vi "ModuloTeste.vi"(0 "IA State Input":T3, 1 "atacando ao contrário?":bool=TRUE, 3 "test module":T1) -> (14 "IA State Output":T3, 15 "ball":dbl(graph), 17 "Robot":dbl(graph))   [LabVIEW 2017]
uses:
  Core/AI Input.ctl
  Core/AI Robot.ctl
  Functions Enum.ctl
  AttackerStates.ctl
  Path Planning/RRT/PathDests.ctl
  Path Planning/RRT/PathDest.ctl
  Core/AI Ball.ctl
  Core/Field Size.ctl
  Core/AI Judge.ctl
  Command Enum.ctl
  Util/Events/Events.ctl
  Test/TestModule.ctl
  Util/Select None or Robot.ctl
  <vilib>/Analysis/_algsub.llb/Real Vector Norm.vi
  <vilib>/Analysis/NI_AALPro.lvlib
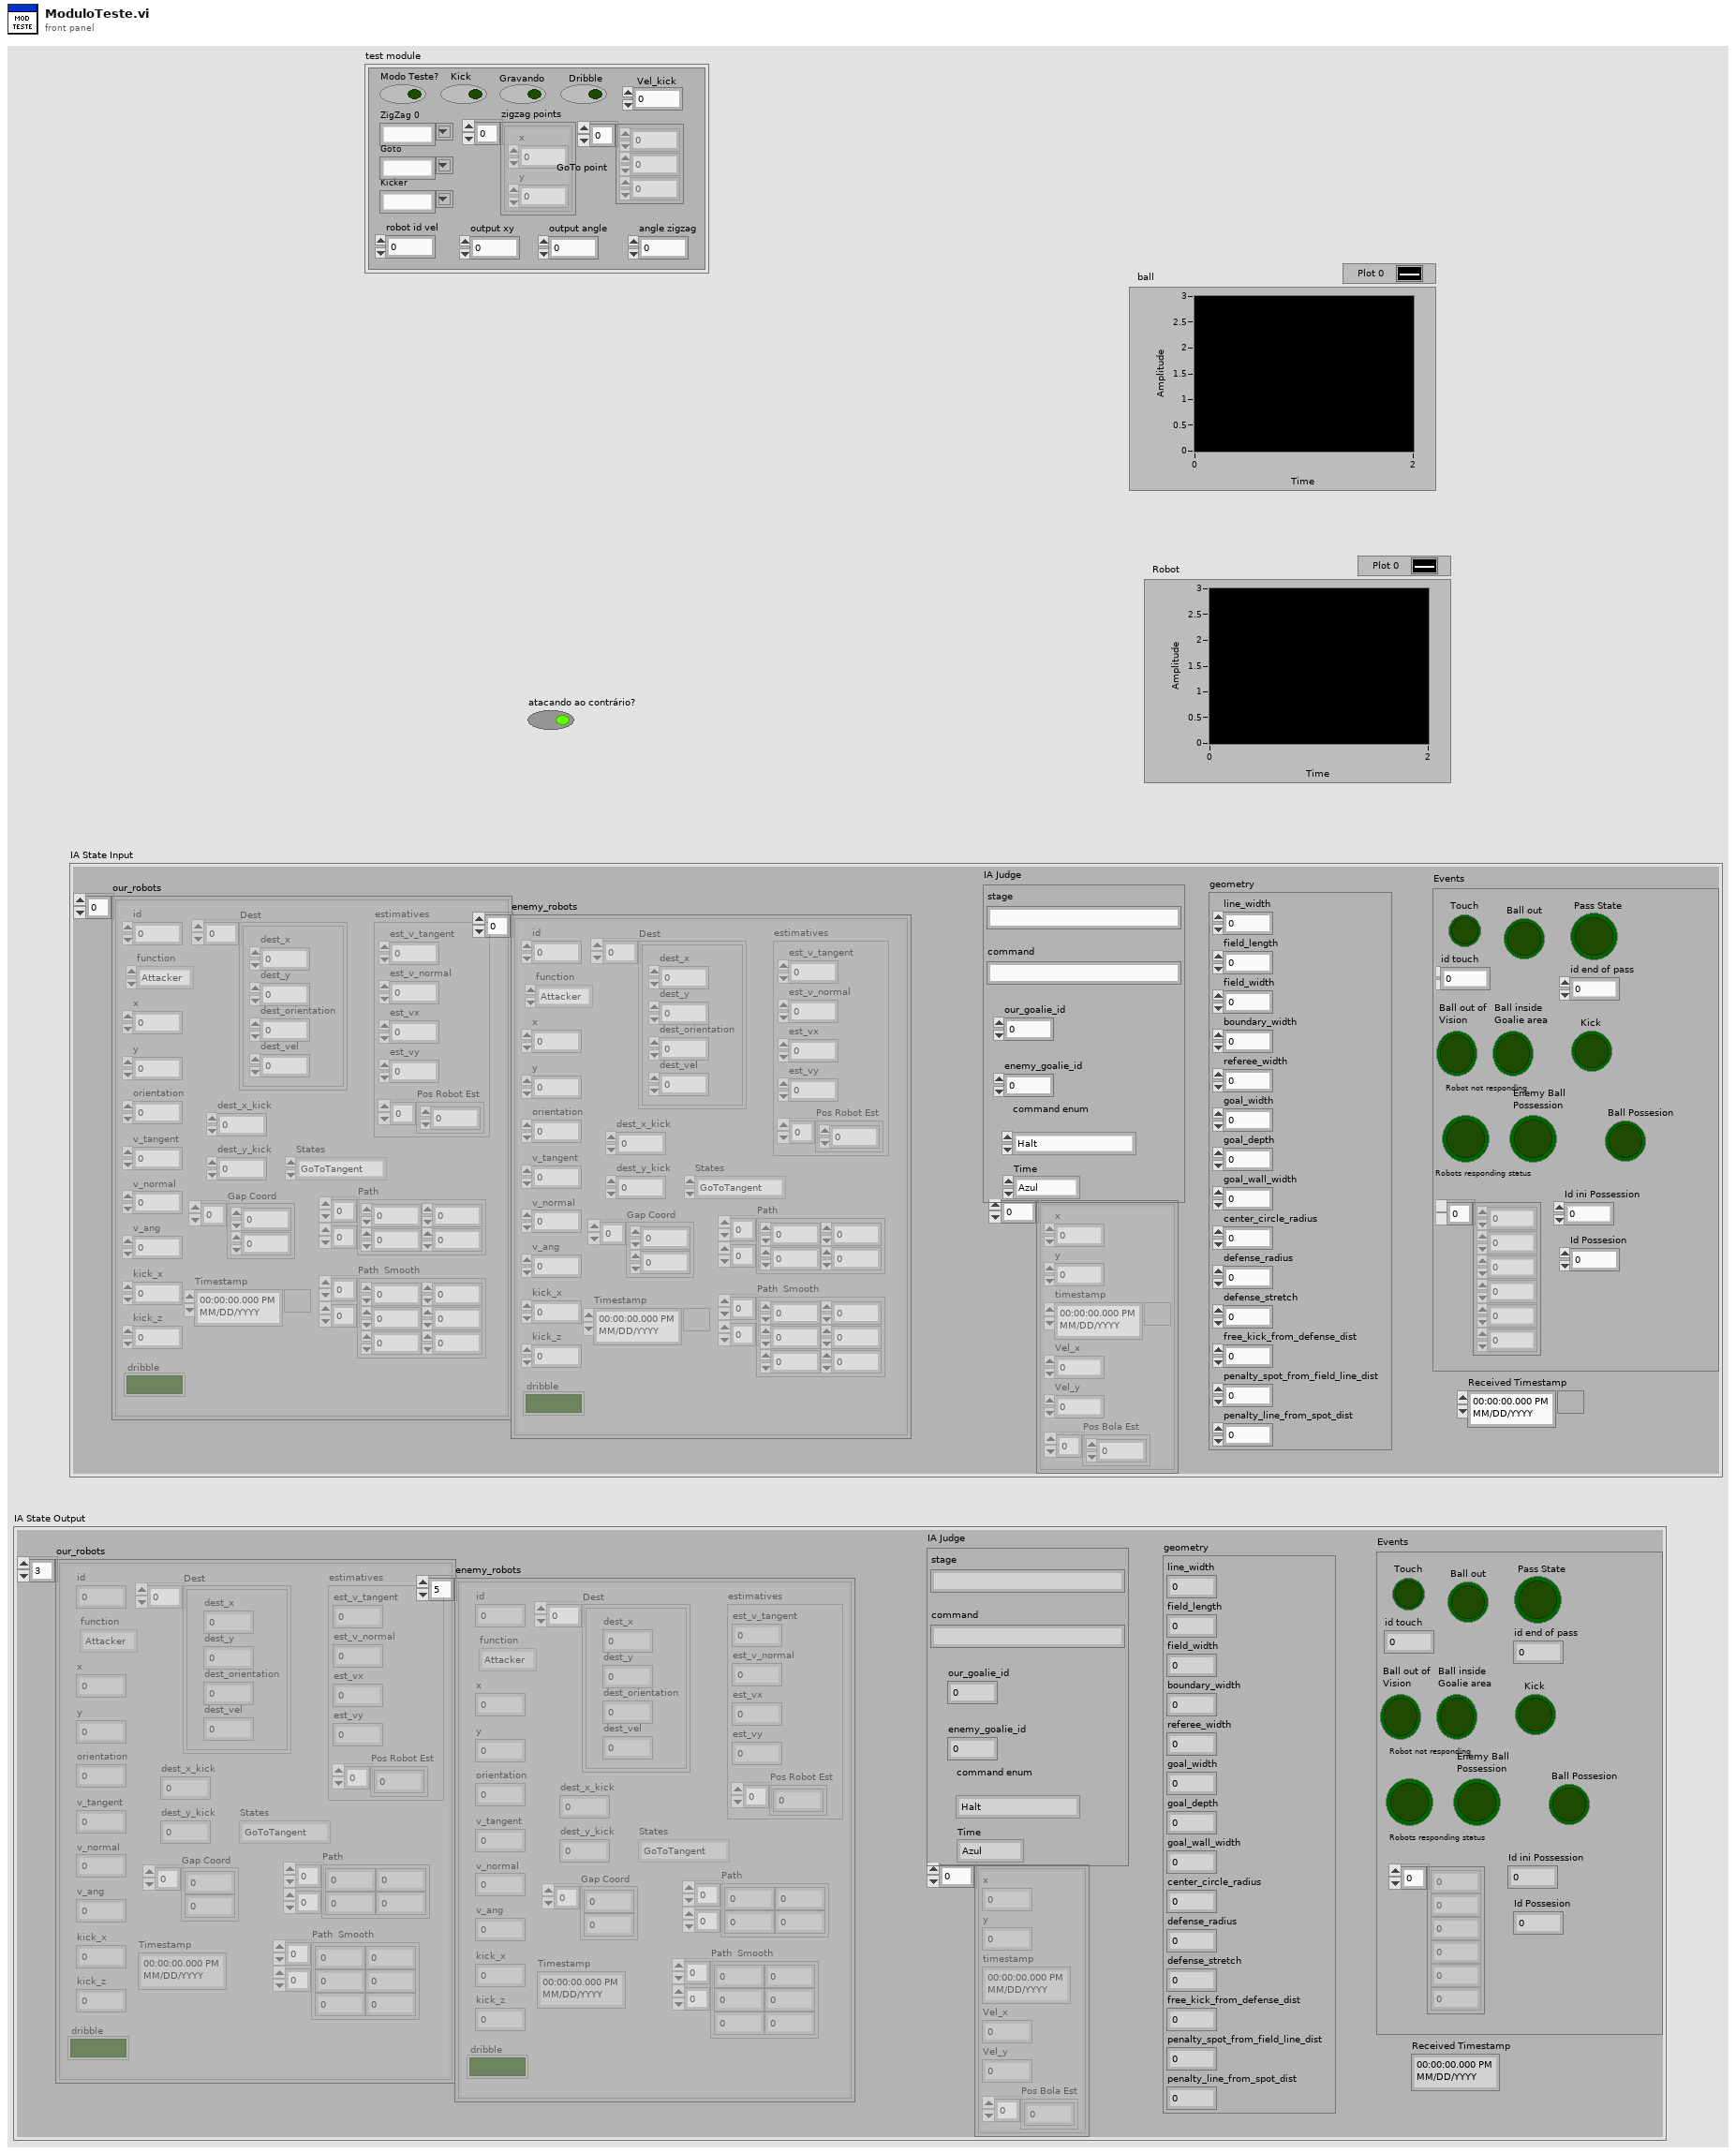
[diagram p1: front panel]
types:
  T1 = typedef "TestModule.ctl" = cluster{"Goto":T2, "ZigZag 0":T2, "Kicker":T2, "Vel_kick":dbl, "Kick":bool, "Modo Teste?":bool, "GoTo point":dbl[], "zigzag points":cluster{"x":dbl, "y":dbl}[], "robot id vel":u32, "Dribble":bool, "Gravando":bool, "output xy":dbl, "output angle":dbl, "angle zigzag":dbl}
  T2 = typedef "Select None or Robot.ctl" = string
  T3 = typedef "AI Input.ctl" = cluster{"our_robots":T4[], "enemy_robots":T4[], "balls":T9[], "geometry":T10, "IA Judge":T11, "Received Timestamp":timestamp, "Events":T13}
  T4 = typedef "AI Robot.ctl" = cluster{"id":u32, "function":T5, "x":dbl, "y":dbl, "orientation":dbl, "v_tangent":dbl, "v_normal":dbl, "v_ang":dbl, "kick_x":dbl, "kick_z":dbl, "dribble":bool, "Timestamp":timestamp, "estimatives":cluster{"est_v_tangent":dbl, "est_v_normal":dbl, "est_vx":dbl, "est_vy":dbl, "Pos Robot Est":dbl[]}, "dest_x_kick":dbl, "dest_y_kick":dbl, "Gap Coord":dbl[], "States":T6, "Path ":dbl[][], "Path  Smooth":dbl[][], "Dest":T7}
  T5 = typedef "Functions Enum.ctl" = enum16{"Attacker", "Goalie", "Defender", "Striker", "Goto 0", "Dummy", "Kicker", "ZigZag"}
  T6 = typedef "AttackerStates.ctl" = enum16{"Pass", "GoToTangent", "BallGetting", "GoToKick", ""}
  T7 = typedef "PathDests.ctl" = T8[]
  T8 = typedef "PathDest.ctl" = cluster{"dest_x":dbl, "dest_y":dbl, "dest_orientation":dbl, "dest_vel":dbl}
  T9 = typedef "AI Ball.ctl" = cluster{"x":dbl, "y":dbl, "timestamp":timestamp, "Vel_x":dbl, "Vel_y":dbl, "Pos Bola Est":dbl[]}
  T10 = typedef "Field Size.ctl" = cluster{"line_width":u32, "field_length":u32, "field_width":u32, "boundary_width":u32, "referee_width":u32, "goal_width":u32, "goal_depth":u32, "goal_wall_width":u32, "center_circle_radius":u32, "defense_radius":u32, "defense_stretch":u32, "free_kick_from_defense_dist":u32, "penalty_spot_from_field_line_dist":u32, "penalty_line_from_spot_dist":u32}
  T11 = typedef "AI Judge.ctl" = cluster{"stage":string, "command":string, "our_goalie_id":dbl, "enemy_goalie_id":dbl, "command enum":T12, "Time":enum16{"Azul", "Amarelo"}}
  T12 = typedef "Command Enum.ctl" = enum16{"Halt", "Stop", "Force Start", "PKA Normal Start", "Prepare Kickoff Ally", "PKE Normal Start", "Prepare Kickoff Enemy", "Prepare Penalty Ally", "PPA Normal Start", "Prepare Penalty Enemy", "PPE Normal Start", "Direct Free Enemy", "Direct Free Ally", "Indirect Free Enemy", "Indirect Free Ally", "Timeout Enemy", "Timeout Ally", "Goal Enemy", "Goal Ally", "Ball Placement Enemy", "Ball Placement Ally", "Normal Half Time", "Extra Time Break", "Extra Half Time", "None", "Post Game"}
  T13 = typedef "Events.ctl" = cluster{"Touch":bool, "Ball out":bool, "id touch":dbl, "Ball out of \nVision":bool, "Ball inside \nGoalie area":bool, "Robot not responding":bool, "Robots responding status":dbl[], "Enemy Ball \nPossession":bool, "Pass State":bool, "id end of pass":dbl, "Kick":bool, "Id ini Possession":dbl, "Ball Possesion":bool, "Id Possesion":dbl}
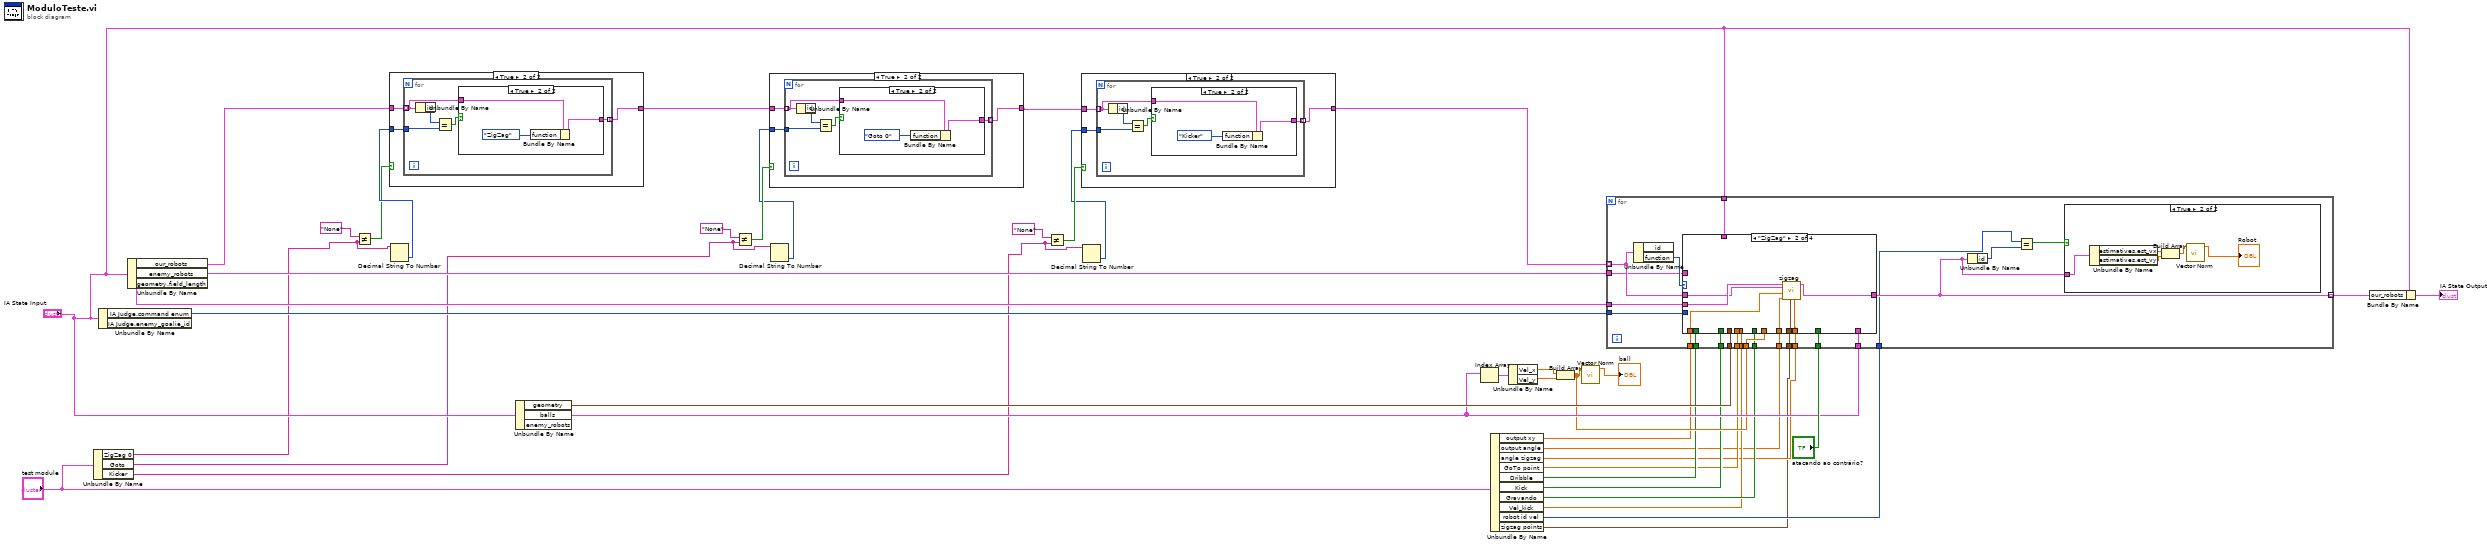
[diagram p0: block diagram]
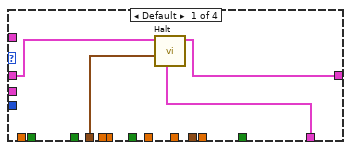
[diagram p9: hidden frame]
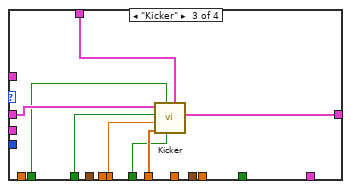
[diagram p10: hidden frame]
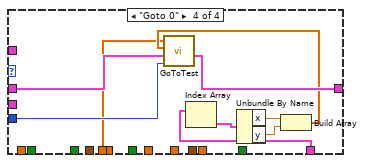
[diagram p11: hidden frame]
diagram:
  n1 = Unbundle By Name("test module") -> ("ZigZag 0"=w14:T2, "Goto"=w13:T2, "Kicker"=w12:T2)
  n2 = Unbundle By Name("IA State Input") -> ("IA Judge.command enum"=w40:T12)  [unwired: 1 out]
  n3 = Unbundle By Name("IA State Input") -> ("our_robots"=w31:T4[], "enemy_robots"=w36:T4[])  [unwired: 1 out]
  n4 = Not Equal?(x="None", y=w14) -> (x != y?=w33:bool)
  n5 = Decimal String To Number(string=w14) -> (number=w34:i32)  [unwired: 2 in, 1 out]
  n6 = case shown="True" w33 {
    tunnel: w34 -> [_ w44]
    tunnel: [w41 w43] -> w28
    tunnel: w31 -> [w41 w42]
    frame False {
    }
    frame True {
      n7 = for {
        tunnel: w44 -> [w48]
        tunnel: [w46] -> w43 mode=indexing
        tunnel: w42 -> [w45] mode=indexing
        n8 = Unbundle By Name(w45) -> ("id"=w49:u32)
        n9 = Equal?(x=w49, y=w48) -> (x = y?=w47:bool)
        n10 = case shown="True" w47 {
          tunnel: [w50 w53] -> w46
          tunnel: w45 -> [w50 w51]
          frame False {
          }
          frame True {
            n11 = Bundle By Name(cluster=w51, "function"=Functions_Enum."ZigZag") -> (w53:T4)
          }
        }
      }
    }
  }
  n12 = Unbundle By Name("IA State Input") -> ("geometry"=w37:T10, "balls"=w21:T9[])  [unwired: 1 out]
  n13 = Not Equal?(x="None", y=w13) -> (x != y?=w30:bool)
  n14 = Decimal String To Number(string=w13) -> (number=w27:i32)  [unwired: 2 in, 1 out]
  n15 = case shown="True" w30 {
    tunnel: w27 -> [_ w57]
    tunnel: [w54 w56] -> w23
    tunnel: w28 -> [w54 w55]
    frame False {
    }
    frame True {
      n16 = for {
        tunnel: w57 -> [w61]
        tunnel: [w59] -> w56 mode=indexing
        tunnel: w55 -> [w58] mode=indexing
        n17 = Unbundle By Name(w58) -> ("id"=w62:u32)
        n18 = Equal?(x=w62, y=w61) -> (x = y?=w60:bool)
        n19 = case shown="True" w60 {
          tunnel: [w63 w66] -> w59
          tunnel: w58 -> [w63 w64]
          frame False {
          }
          frame True {
            n20 = Bundle By Name(cluster=w64, "function"=Functions_Enum."Goto 0") -> (w66:T4)
          }
        }
      }
    }
  }
  n21 = Not Equal?(x="None", y=w12) -> (x != y?=w26:bool)
  n22 = Decimal String To Number(string=w12) -> (number=w24:i32)  [unwired: 2 in, 1 out]
  n23 = case shown="True" w26 {
    tunnel: w24 -> [_ w70]
    tunnel: [w67 w69] -> w22
    tunnel: w23 -> [w67 w68]
    frame False {
    }
    frame True {
      n24 = for {
        tunnel: w70 -> [w74]
        tunnel: [w72] -> w69 mode=indexing
        tunnel: w68 -> [w71] mode=indexing
        n25 = Unbundle By Name(w71) -> ("id"=w75:u32)
        n26 = Equal?(x=w75, y=w74) -> (x = y?=w73:bool)
        n27 = case shown="True" w73 {
          tunnel: [w76 w79] -> w72
          tunnel: w71 -> [w76 w77]
          frame False {
          }
          frame True {
            n28 = Bundle By Name(cluster=w77, "function"=Functions_Enum."Kicker") -> (w79:T4)
          }
        }
      }
    }
  }
  n29 = Index Array(array=w21) -> (element=w20:T9)  [unwired: 1 in]
  n30 = Unbundle By Name("test module") -> ("output xy"=w4:dbl, "output angle"=w3:dbl, "angle zigzag"=w2:dbl, "GoTo point"=w5:dbl[], "Dribble"=w10:bool, "Kick"=w9:bool, "Gravando"=w8:bool, "Vel_kick"=w7:dbl, "robot id vel"=w6:u32, "zigzag points"=w1:cluster{"x":dbl, "y":dbl}[])
  n31 = Unbundle By Name(w20) -> ("Vel_x"=w19:dbl, "Vel_y"=w18:dbl)
  n32 = Build Array(w19, w18) -> (w16:dbl[])
  n33 = call-poly <vilib>:"Vector Norm.vi"("Input Vector"=w16) -> ("norm"=→"ball":dbl)  [unwired: 9 in, 1 out]
  n34 = for {
    tunnel: w22 -> [w101] mode=indexing
    tunnel: [w92] -> w39 mode=indexing
    tunnel: w40 -> [w100]
    tunnel: "IA State Input" -> [w99]
    tunnel: w37 -> [w98]
    tunnel: w21 -> [w97]
    tunnel: w36 -> [w96]
    tunnel: "atacando ao contrário?" -> [w95]
    tunnel: w1 -> [w91]
    tunnel: w16 -> [w90]
    tunnel: "IA State Input" -> [w89]
    tunnel: w10 -> [w88]
    tunnel: w9 -> [w87]
    tunnel: w8 -> [w86]
    tunnel: w7 -> [w85]
    tunnel: w6 -> [w84]
    tunnel: w5 -> [w83]
    tunnel: w4 -> [w82]
    tunnel: w3 -> [w81]
    tunnel: w2 -> [w80]
    n35 = Unbundle By Name(w101) -> ("function"=w102:T5)  [unwired: 1 out]
    n36 = case shown="\"ZigZag\"" w102 {
      tunnel: w101 -> [w111 w116 w125 w135]
      tunnel: [w110 w118 w126 w134] -> w92
      tunnel: w100 -> [_ _ _ w133]
      tunnel: w99 -> [_ w117 _ _]
      tunnel: w98 -> [w109 _ _ _]
      tunnel: w97 -> [w108 _ _ w132]
      tunnel: w96 -> [_ _ _ _]
      tunnel: w95 -> [_ _ _ _]
      tunnel: w91 -> [_ w115 _ _]
      tunnel: w90 -> [_ _ w124 _]
      tunnel: w89 -> [_ _ w123 _]
      tunnel: w88 -> [_ _ w122 _]
      tunnel: w87 -> [_ _ w121 _]
      tunnel: w86 -> [_ _ w120 _]
      tunnel: w85 -> [_ _ w119 _]
      tunnel: w83 -> [_ _ _ w127]
      tunnel: w82 -> [_ w114 _ _]
      tunnel: w81 -> [_ w113 _ _]
      tunnel: w80 -> [_ w112 _ _]
      frame Default {
        n37 = call "Halt.vi"("balls"=w108, "Field Size in"=w109, "Robot in"=w111) -> ("Robot out"=w110:T4)  [unwired: 8 in]
      }
      frame "ZigZag" {
        n38 = call "zigzag.vi"("angulo"=w112, "points 3"=w115, "output angle"=w113, "output xy"=w114, "Current Robot"=w116, "Al Input"=w117) -> ("Output Robot"=w118:T4)  [unwired: 5 in]
      }
      frame "Kicker" {
        n39 = call "Kicker.vi"("IA State Input"=w123, "gravar"=w120, "Dribble"=w122, "Ball velocity"=w124, "Vel_kick"=w119, "Kick?"=w121, "Robot in"=w125) -> ("output cluster"=w126:T4)  [unwired: 4 in]
      }
      frame "Goto 0" {
        n40 = Index Array(array=w132) -> (element=w131:T9)  [unwired: 1 in]
        n41 = Unbundle By Name(w131) -> ("x"=w130:dbl, "y"=w129:dbl)
        n42 = Build Array(w130, w129) -> (w128:dbl[])
        n43 = call "GoToTest.vi"("command\nenum"=w133, "Robot In"=w135, "Ball"=w128, "GoTo point"=w127) -> ("Robot Out"=w134:T4)  [unwired: 7 in]
      }
    }
    n44 = Unbundle By Name(w92) -> ("id"=w94:u32)
    n45 = Equal?(x=w84, y=w94) -> (x = y?=w93:bool)
    n46 = case shown="True" w93 {
      tunnel: w92 -> [_ w107]
      frame False {
      }
      frame True {
        n47 = Unbundle By Name(w107) -> ("estimatives.est_vx"=w106:dbl, "estimatives.est_vy"=w105:dbl)
        n48 = Build Array(w106, w105) -> (w104:dbl[])
        n49 = call-poly <vilib>:"Vector Norm.vi"("Input Vector"=w104) -> ("norm"=→"Robot":dbl)  [unwired: 9 in, 1 out]
      }
    }
  }
  n50 = Bundle By Name(cluster="IA State Input", "our_robots"=w39) -> (→"IA State Output":T3)
